vi "log process.vi"() -> ()   [LabVIEW 2019]
panel:
  out "rt queue":refnum<queue>
  out "data":refnum<queue>
  out "error out":errorcluster
  out "log":string
  out "path":path
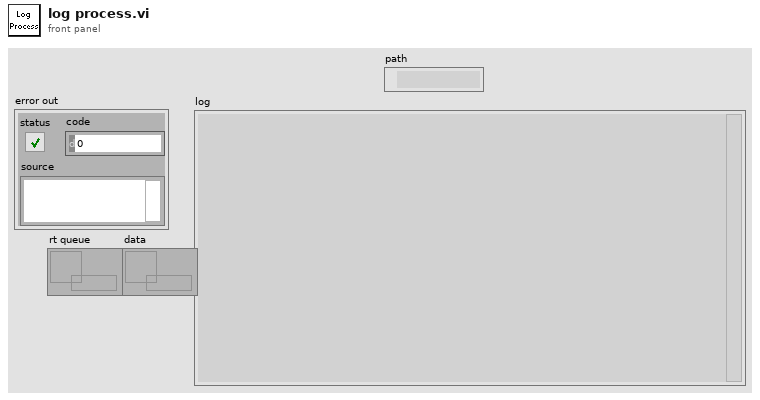
[diagram p1: front panel]
types:
  T1 = enum16{"open", "replace", "create", "open or create", "replace or create", "replace or create with confirmation"}
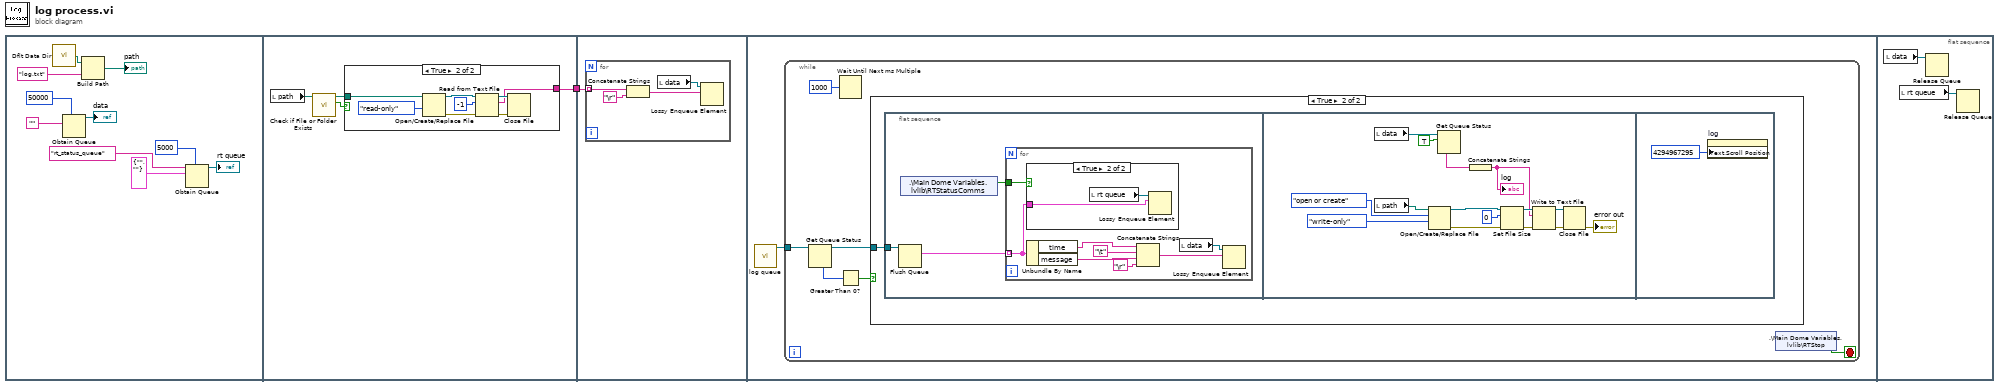
[diagram p0: block diagram]
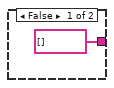
[diagram p2: hidden frame]
diagram:
  n1 = flat-sequence {
    tunnel: [w12] -> w1
    tunnel: w1 -> [w25]
    frame #0 {
      n2 = call <vilib>:"Dflt Data Dir.vi"() -> ("App:Default Data Directory"=w10:path)
      n3 = Obtain Queue(max queue size (-1, unlimited)=50000, element data type="") -> (queue out=→"data":refnum<queue>)  [unwired: 3 in, 2 out]
      n4 = Build Path(base path=w10, name or relative path="log.txt") -> (appended path=→"path":path)
      n5 = Obtain Queue(max queue size (-1, unlimited)=5000, name (unnamed)="rt_status_queue", element data type=cluster{"time":string, "message":string} {"time"="", "message"=""}) -> (queue out=→"rt queue":refnum<queue>)  [unwired: 2 in, 2 out]
    }
    frame #1 {
      n6 = local read "path"() -> (w15:path)
      n7 = call <vilib>:"Check if File or Folder Exists.vi"("path"=w15) -> ("file or folder exists?"=w14:bool, "dup path"=w13:path)  [unwired: 8 in, 1 out]
      n8 = case shown="True" w14 {
        tunnel: w13 -> [_ w24]
        tunnel: [string[] [] w17] -> w12
        frame False {
        }
        frame True {
          n9 = Open/Create/Replace File(file path (use dialog)=w24, access (0:read/write)=enum16{"read/write", "read-only", "write-only"}."read-only") -> (refnum out=w21:refnum<file>, error out=w20:errorcluster)  [unwired: 4 in, 1 out]
          n10 = Read from Text File(file (use dialog)=w21, count=-1, error in=w20) -> (refnum out=w19:refnum<file>, text=w17:string[], error out=w18:errorcluster)  [unwired: 1 in, 1 out]
          n11 = Close File(refnum=w19, error in=w18) -> ()  [unwired: 2 out]
        }
      }
    }
    frame #2 {
      n12 = for {
        tunnel: w25 -> [w29] mode=indexing
        n13 = Concatenate Strings(w29, "\r") -> (w26:string)
        n14 = local read "data"() -> (w27:refnum<queue>)
        n15 = Lossy Enqueue Element(queue=w27, element=w26) -> ()  [unwired: 1 in, 4 out]
      }
    }
    frame #3 {
      n16 = call "log queue.vi"() -> ("queue out"=w30:refnum<queue>)  [unwired: 11 in]
      n17 = while {
        tunnel: w30 -> [w36]
        stop <- w31 stop-if-true
        n18 = Get Queue Status(queue=w36) -> (queue out=w33:refnum<queue>, # elements in queue=w35:i32)  [unwired: 2 in, 6 out]
        n19 = Wait Until Next ms Multiple(millisecond multiple=u32 1000) -> ()  [unwired: 1 out]
        n20 = Greater Than 0?(x=w35) -> (x > 0?=w34:bool)
        n21 = case shown="True" w34 {
          tunnel: w33 -> [_ w37]
          frame False {
          }
          frame True {
            n22 = flat-sequence {
              tunnel: w37 -> [w40]
              frame #0 {
                n23 = Flush Queue(queue=w40) -> (remaining elements=w39:cluster{"time":string, "message":string}[])  [unwired: 1 in, 2 out]
                n24 = shared-variable ".\\Main Dome Variables.lvlib\\RTStatusComms"() -> (w38:bool)  [unwired: 1 in, 1 out]
                n25 = for {
                  tunnel: w39 -> [w42] mode=indexing
                  tunnel: w38 -> [w41]
                  n26 = case shown="True" w41 {
                    tunnel: w42 -> [_ w50]
                    frame False {
                    }
                    frame True {
                      n27 = local read "rt queue"() -> (w49:refnum<queue>)
                      n28 = Lossy Enqueue Element(queue=w49, element=w50) -> ()  [unwired: 1 in, 4 out]
                    }
                  }
                  n29 = Unbundle By Name(w42) -> ("time"=w45:string, "message"=w46:string)
                  n30 = Concatenate Strings(w45, "\t", w46, "\r") -> (w43:string)
                  n31 = local read "data"() -> (w44:refnum<queue>)
                  n32 = Lossy Enqueue Element(queue=w44, element=w43) -> ()  [unwired: 1 in, 4 out]
                }
              }
              frame #1 {
                n33 = local read "data"() -> (w53:refnum<queue>)
                n34 = local read "path"() -> (w65:path)
                n35 = Open/Create/Replace File(file path (use dialog)=w65, operation (0:open)=T1."open or create", access (0:read/write)=enum16{"read/write", "read-only", "write-only"}."write-only") -> (refnum out=w60:refnum<file>, error out=w62:errorcluster)  [unwired: 3 in, 1 out]
                n36 = Get Queue Status(queue=w53, return elements? (F)=TRUE) -> (elements=w52:string[])  [unwired: 1 in, 7 out]
                n37 = Concatenate Strings(w52) -> (w57:string)
                "log" <- w57
                n38 = Set File Size(4:w62, 6:i64 0 ("size (in bytes)"), 7:w60) -> (0:w59:errorcluster, 3:w58:refnum<file>)
                n39 = Write to Text File(file (use dialog)=w58, text=w57, error in=w59) -> (refnum out=w56:refnum<file>, error out=w55:errorcluster)  [unwired: 1 in, 1 out]
                n40 = Close File(refnum=w56, error in=w55) -> (error out=→"error out":errorcluster)  [unwired: 1 out]
              }
              frame #2 {
                n41 = property on="log" class="Str"("Text.Scroll Position"=u32 4294967295) -> ()  [unwired: 2 in, 2 out]
              }
            }
          }
        }
        n42 = shared-variable ".\\Main Dome Variables.lvlib\\RTStop"() -> (w31:bool)  [unwired: 1 in, 1 out]
      }
    }
    frame #4 {
      n43 = local read "data"() -> (w68:refnum<queue>)
      n44 = local read "rt queue"() -> (w67:refnum<queue>)
      n45 = Release Queue(queue=w68) -> ()  [unwired: 2 in, 3 out]
      n46 = Release Queue(queue=w67) -> ()  [unwired: 2 in, 3 out]
    }
  }
